vi "GetAngle90.vi"() -> ()   [LabVIEW 2016, in "Gear Manipulator.lvclass"]
uses:
  Gear Manipulator.lvclass
panel:
  out "Gear Manipulator.lvclass":refnum<class "Gear Manipulator.lvclass">
  in  "Gear Manipulator.lvclass":refnum<class "Gear Manipulator.lvclass">
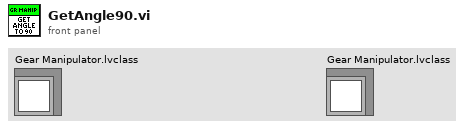
[diagram p1: front panel]
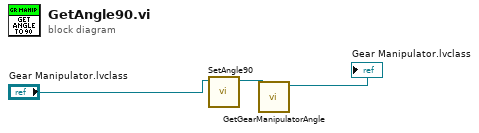
[diagram p0: block diagram]
diagram:
  n1 = call "SetAngle90.vi"("Gear Manipulator.lvclass"="Gear Manipulator.lvclass") -> ("Gear Manipulator.lvclass"=w2:refnum<class "Gear Manipulator.lvclass">)  [unwired: 10 in]
  n2 = call "GetGearManipulatorAngle.vi"("Gear Manipulator in"=w2) -> ("Gear Manipulator out"=→"Gear Manipulator.lvclass":refnum<class "Gear Manipulator.lvclass">)  [unwired: 9 in, 1 out]
